vi "Get Module Node from Identifier.vi"(8 "error in":errorcluster, 10 "module identifier":string, 11 "routing and faulting in":T1 format="%.0x") -> (0 "error out":errorcluster, 1 "found":bool, 2 "module node":T1 format="%.0x", 3 "routing and faulting out":T1 format="%.0x")   [LabVIEW 2020, in "Routing and Faulting Scripting.lvlib"]
uses:
  Routing and Faulting Scripting.lvlib
  <vilib>/NI VeriStand/Custom Device API/Custom Device Item Ref.ctl
  NationalInstruments.VeriStand.SystemStorage
  <vilib>/NI VeriStand/Custom Device API/Custom Device API.lvlib
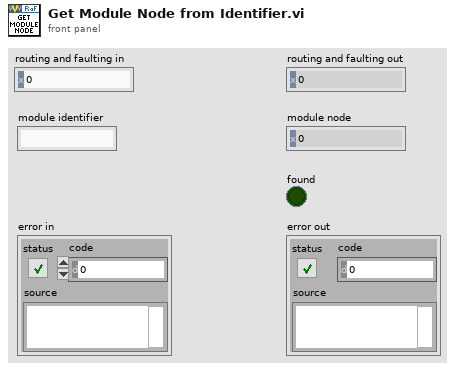
[diagram p1: front panel]
types:
  T1 = typedef "Custom Device API.lvlib/Custom Device Item Ref.ctl" = u64
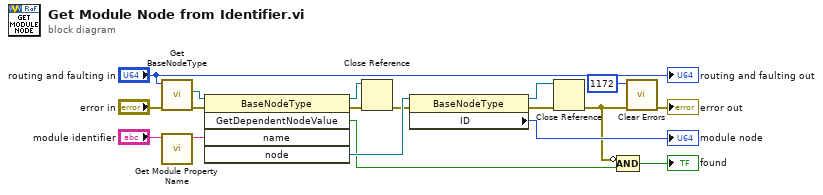
[diagram p0: block diagram]
diagram:
  n1 = call "Get BaseNodeType.vi"("error in"="error in", "item in"="routing and faulting in") -> ("error out"=w14:errorcluster, "BaseNodeType"=w13:refnum<k24>)  [unwired: 7 in, 1 out]
  n2 = call "Get Module Property Name.vi"("module identifier"="module identifier") -> ("module property name"=w18:string)  [unwired: 10 in]
  n3 = invoke class="BaseNodeType" method="GetDependentNodeValue"(reference=w13, error in=w14, "name"=w18) -> (reference out=w11:refnum<k24>, error out=w16:errorcluster, "GetDependentNodeValue"=w5:bool, "node"=w10:refnum<k24>)  [unwired: 2 in, 1 out]
  n4 = Close Reference(reference=w11, error in (no error)=w16) -> (error out=w6:errorcluster)
  n5 = property class="BaseNodeType"(reference=w10, error in=w6) -> (reference out=w8:refnum<k24>, error out=w9:errorcluster, "ID"=→"module node":u64)
  n6 = Close Reference(reference=w8, error in (no error)=w9) -> (error out=w4:errorcluster)
  n7 = Compound Arithmetic op=AND(invert w4, w5) -> (→"found":bool)
  n8 = call <vilib>:"Clear Errors.vi"("error in (no error)"=w4, "specific error code to clear (0: all)"=1172) -> ("error out"=→"error out":errorcluster)  [unwired: 4 in, 1 out]
  "routing and faulting out" <- "routing and faulting in"
